vi "FP_Size Using Position and Bounds.vi"(6 "Border Spacing":i16, 8 "Error":errorcluster, 9 "Bounds":T3, 10 "Position":T2, 11 "VI":refnum<vi>) -> (0 "Error Out":errorcluster, 2 "Front Panel Box Out":T1, 3 "VI Out":refnum<vi>)   [LabVIEW 2016]
uses:
  <vilib>/Utility/miscctls.llb/LVBoundsTypeDef.ctl
  <vilib>/Utility/miscctls.llb/LVPositionTypeDef.ctl
  <vilib>/Utility/miscctls.llb/LVRectTypeDef.ctl
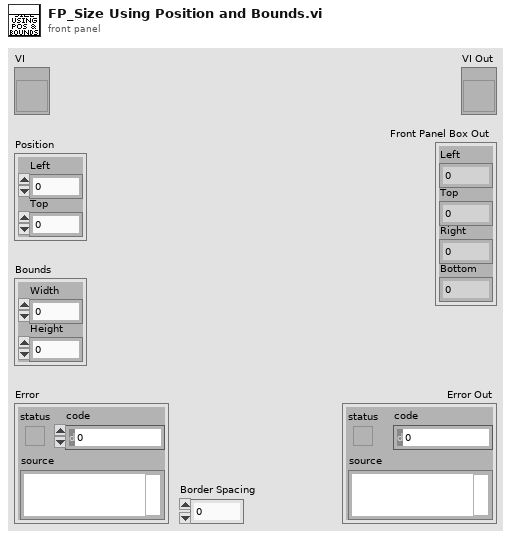
[diagram p1: front panel]
types:
  T1 = typedef "LVRectTypeDef.ctl" = cluster{"Left":i16, "Top":i16, "Right":i16, "Bottom":i16}
  T2 = typedef "LVPositionTypeDef.ctl" = cluster{"Left":i32, "Top":i32}
  T3 = typedef "LVBoundsTypeDef.ctl" = cluster{"Width":u32, "Height":u32}
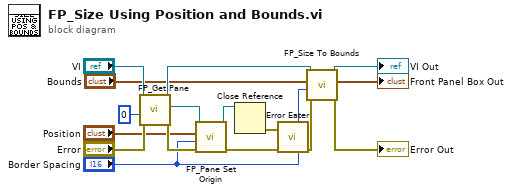
[diagram p0: block diagram]
diagram:
  n1 = call "FP_Get Pane.vi"("Error"="Error", "Pane Index"=0, "VI"="VI") -> ("Error Out"=w14:errorcluster, "Pane Refnum Out"=w15:refnum<vi>, "VI Out"=w11:refnum<vi>)  [unwired: 6 in]
  n2 = call "FP_Pane Set Origin.vi"("Error"=w14, "Border Spacing"="Border Spacing", "FP Position"="Position", "Pane"=w15) -> ("Error Out"=w7:errorcluster, "Pane In Out"=w10:refnum<vi>)  [unwired: 6 in]
  n3 = Close Reference(reference=w10) -> (error out=w1:errorcluster)  [unwired: 1 in]
  n4 = call "Error Eater.vi"("error in (no error)"=w1) -> ()  [unwired: 2 in]
  n5 = call "FP_Size To Bounds.vi"("Error"=w7, "Border Spacing"="Border Spacing", "Bounds"="Bounds", "VI"=w11) -> ("Error Out"=→"Error Out":errorcluster, "Front Panel box"=→"Front Panel Box Out":T1, "VI Out"=→"VI Out":refnum<vi>)  [unwired: 5 in]
